vi "StringToU8.vi"(7 "Required size (-1)":i32=-1, 8 "error in (no error)":errorcluster, 11 "HEX text in":string) -> (0 "error out":errorcluster, 3 "ArrayU8 out":u8[](array[numeric]) format="%02x")   [LabVIEW 2012, in "Encryption.lvlib"]
doc: "This VI converts an ASCII HEX string (ascii values 0-f) into an array of U8."
uses:
  Encryption.lvlib
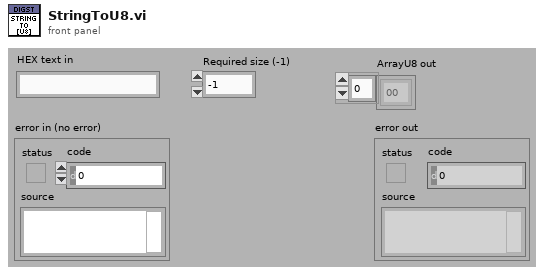
[diagram p1: front panel]
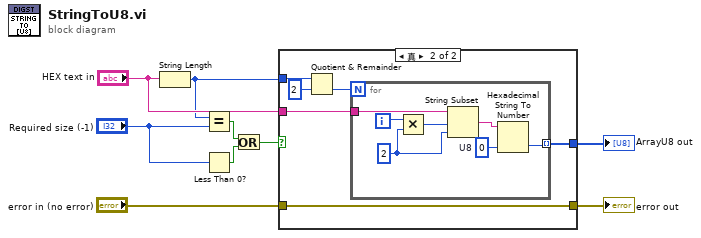
[diagram p0: block diagram]
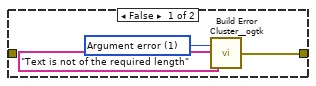
[diagram p2: hidden frame]
diagram:
  n1 = String Length(string="HEX text in") -> (length=w7:i32)
  n2 = Equal?(x=w7, y="Required size (-1)") -> (x = y?=w5:bool)
  n3 = Less Than 0?(x="Required size (-1)") -> (x < 0?=w4:bool)
  n4 = Or(x=w5, y=w4) -> (x .or. y?=w3:bool)
  n5 = case shown="真" w3 {
    tunnel: w7 -> [_ w18]
    tunnel: "HEX text in" -> [_ w15]
    tunnel: [_ w14] -> w8
    tunnel: [w12 w13] -> w2
    tunnel: "error in (no error)" -> [_ w13]
    frame False {
      w11 = 1 items=["No error", "Argument error", "Memory is full", "Out of zone", "End of file", "File already open", "Generic file I/O error", "File not found", "File permission error", "Disk is full", "Duplicate path", "Too many files open", "System feature not enabled", "Resource file not found", "Cannot add resource", "Resource not found", "Image not found", "Image memory error", "Pen does not exist", "Config type invalid", "Config token not found", "Config parse error", "Config memory error", "Bad external code format", "Bad external code offset", "External code not present", "Null window", "Destroy window error", "Null menu", "Print aborted", "Bad print record", "Print driver error", "Windows error during printing", "Memory error during printing", "Print dialog error", "Generic print error", "Invalid device refnum", "Device not found", "Device parameter error", "Device unit error", "Cannot open device", "Device call aborted", "Generic error", "Cancelled by user", "Object ID too low", "Object ID too high", "Object not in heap", "Unknown heap", "Unknown object (invalid DefProc)", "Unknown object (DefProc not in table)", "Message out of range", "Invalid (null) method", "Unknown message", "Manager call not supported", "Bad address", "Network operation in progress", "Network operation timed out", "Connection is busy", "Network attribute not supported", "Network error", "Address in use", "System out of memory", "Connection aborted", "Connection refused", "Not connected", "Already connected", "Connection closed", "Initialization error (interapplication manager)", "Bad occurrence", "Wait on unbound occurrence handler", "Occurrence queue overflow", "Datalog type conflict", "Unused", "Unrecognized type (interapplication manager)", "Memory corrupt", "Failed to make temporary DLL", "Old CIN version", "Drag socket not found", "Failed to load drop-object", "Failed to register OLE object", "Failed to release OLE object", "Format specifier type mismatch", "Unknown format specifier", "Too few format specifiers", "Too many format specifiers", "Scan failed", "Newer CIN version", "Error converting to variant", "Runtime menu error", "Password tampered", "Variant attribute not found", "Incompatible variant data type", "Event data is not available", "Event Store is not present", "Occurrence is not found", "Event Queue is not created", "Event info is not available", "Refnum passed is NULL", "Error retrieving Class GUID", "Error retrieving CoClass GUID", "Error retrieving TypeLib GUID.", "Bad built application magic bytes.", "Specific driver is different from the specific driver associated with the Logical Name.", "There is no session opened to the class driver.", "Max Error", "MAX - Error with config objects", "MAX - Error loading configuration", "MAX - Group not supported"]
      n6 = call <userlib>:"Build Error Cluster__ogtk.vi"("String to Prepend to source (\"\")"="Text is not of the required length" ("String to Prepend to source (\"\")"), "code"=w11) -> ("error out"=w12:errorcluster)
    }
    frame True {
      n7 = Quotient & Remainder(x=w18, y=2) -> (floor(x/y)=w16:i32)  [unwired: 1 out]
      n8 = for {
        N: w16 -> [_]
        tunnel: w15 -> [w25]
        tunnel: [w19] -> w14 mode=indexing
        i -> [w23]
        w20 = u8 0  # U8
        w22 = 2
        n9 = Multiply(x=w23, y=w22) -> (x*y=w24:i32)
        n10 = String Subset(string=w25, offset (0)=w24, length (rest)=w22) -> (substring=w21:string)
        n11 = Hexadecimal String To Number(string=w21, default (0uL)=w20) -> (number=w19:u8)  [unwired: 1 in, 1 out]
      }
    }
  }
  "ArrayU8 out" <- w8
  "error out" <- w2
